vi "fpga_Resampling (M Class_60Hz).vi"(0 "signal in":fxp<+/-,24,1>, 1 "number of channels":T2=7 items=["1"=1, "2"=2, "3"=3, "4"=4, "5"=5, "6"=6, "7"=7, "8"=8, "9"=9, "10"=10, "11"=11, "12"=12, "13"=13, "14"=14, "15"=15, "16"=16], 2 "Memory In":refnum<k21>="coefROM", 5 "timestamp [s]":fxp<+,64,32> format="%.42g", 7 "reference channel index":u8, 9 "input data valid? (T)":bool=TRUE, 12 "ready for output? (T)":bool=TRUE) -> (4 "resampled data":T1, 10 "output valid":bool, 14 "ready for input":bool, 15 "error":i32)   [LabVIEW 2013, in "NI_EP_PMU_FPGA.lvlib"]
doc: "Converts even-time-spaced voltage and current signals to even-angle-spaced signals by resampling the voltage and current signals using a sampling rate of 50 kHz. The output signals are synchronous to the line frequency with a constant number of samples per cycle."
uses:
  <vilib>/addons/Electrical Power/PMU/NI_EP_PMU_FPGA.lvlib
  <vilib>/addons/Electrical Power/PQ/Resampling/FPGA/subVIs/fpga_NofCH.ctl
  <vilib>/addons/Electrical Power/PQ/Resampling/FPGA/subVIs/fpga_Resampled.ctl
  <vilib>/addons/Electrical Power/PQ/Resampling/FPGA/subVIs/fpga_Typedef Fnom.ctl
  <vilib>/addons/Electrical Power/PQ/Resampling/NI_EP_Resample_FPGA.lvlib
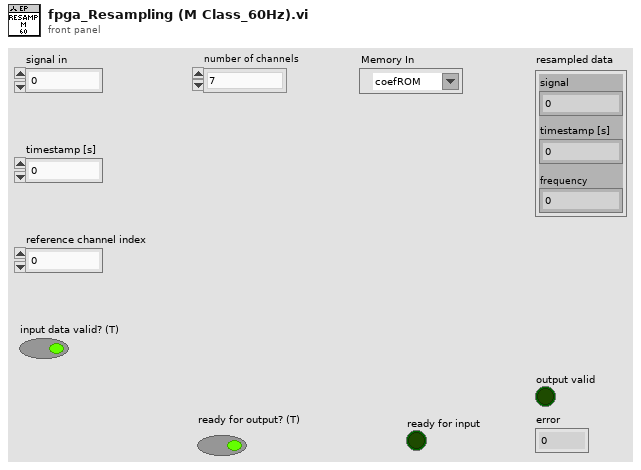
[diagram p1: front panel]
types:
  T1 = typedef "NI_EP_Resample_FPGA.lvlib/fpga_Resampled.ctl" = cluster{"signal":fxp<+/-,32,3>, "timestamp [s]":fxp<+,64,32>, "frequency":fxp<+,32,8>}
  T2 = typedef "NI_EP_Resample_FPGA.lvlib/fpga_NofCH.ctl" = u8
  T3 = typedef "NI_EP_Resample_FPGA.lvlib/fpga_Typedef Fnom.ctl" = u8
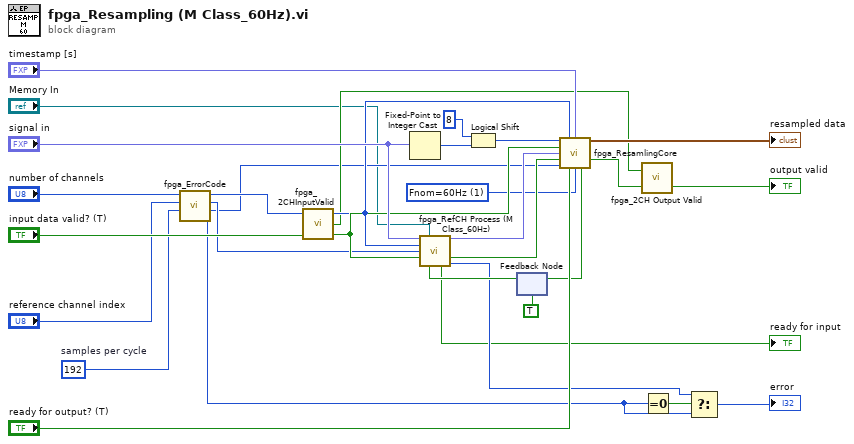
[diagram p0: block diagram]
diagram:
  w7 = u16 192  # samples per cycle
  w11 = T3 1 items=["Fnom=50Hz", "Fnom=60Hz"] ("Fnom")
  n1 = call <vilib>:"fpga_ErrorCode.vi"("samples per cycle"=w7, "reference channel index"="reference channel index", "number of channels"="number of channels") -> ("error"=w4:i32, "samples per cycle out"=w8:u16, "ref channel index out"=w9:u8, "number of CH out"=w10:u8)  [unwired: 5 in]
  n2 = call <vilib>:"fpga_2CHInputValid.vi"("input data valid"="input data valid? (T)", "Channel number"=w10) -> ("input valid"=w21:bool, "1CH?"=w13:bool, "Channel number"=w14:u8)  [unwired: 1 in]
  n3 = Fixed-Point to Integer Cast(1:"signal in") -> (0:w19:i32)
  n4 = Logical Shift(y=i8 8, x=w19) -> (x << y=w17:i32)
  n5 = feedback #1(TRUE ("Ready for reference input")) -> (w20:bool)
  n6 = call <vilib>:"fpga_RefCH Process (M Class_60Hz).vi"("data in <?24.1>"="signal in", "Memory In"="Memory In", "Channel number"=w14, "Reference index"=w9, "input data valid"=w21, "ready for output"=w20) -> ("Filtered Ref data <24,3>"=w16:fxp<+/-,24,3>, "output valid"=w15:bool, "ready for input"=→"ready for input":bool, "error"=w2:i32)  [unwired: 6 in]
  n7 = call <vilib>:"fpga_ResamlingCore.vi"("data in"=w17, "Channel number"=w14, "timestamp"="timestamp [s]", "input data valid"=w21, "reference in"=w16, "input reference valid"=w15, "interpolation factor"=w8, "Ready for output"="ready for output? (T)", "Fnom"=w11) -> ("Resample data and time"=→"resampled data":T1, "output valid"=w12:bool, "Ready for reference input"=w23:bool)  [unwired: 2 in, 2 out]
  n8 = feedback-in #1(w23) -> ()
  n9 = call <vilib>:"fpga_2CH Output Valid.vi"("output valid"=w12, "1CH?"=w13) -> ("output valid"=→"output valid":bool)  [unwired: 1 in]
  n10 = Equal To 0?(x=w4) -> (x = 0?=w5:bool)
  n11 = Select(t=w2, s=w5, f=w4) -> (s? t:f=→"error":i32)
